vi "String-Array zusammenstutzen.vi"(8 "Array":string[](array[string]), 10 "Anzahl Elemente":i32) -> (0 "Array":string[](array[string]))   [LabVIEW 2020, in "AK-Schnittstelle.lvlib"]
uses:
  AK-Schnittstelle.lvlib
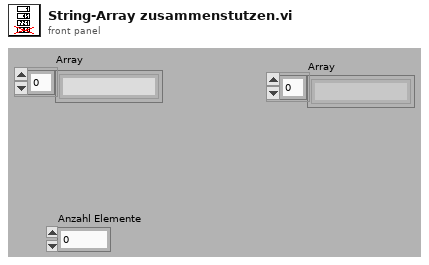
[diagram p1: front panel]
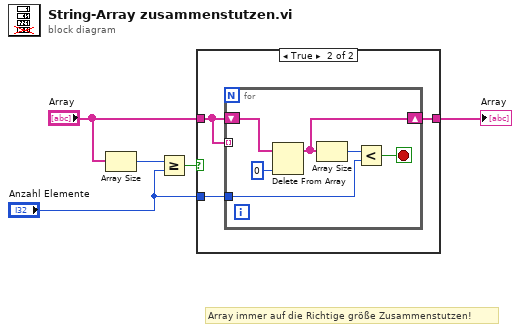
[diagram p0: block diagram]
diagram:
  # "Array immer auf die Richtige größe Zusammenstutzen!"
  n1 = Array Size(array="Array") -> (size(s)=w4:i32)
  n2 = Greater Or Equal?(x=w4, y="Anzahl Elemente") -> (x >= y?=w5:bool)
  n3 = case shown="True" w5 {
    tunnel: "Array" -> [w6 w8]
    tunnel: [w6 w7] -> w1
    tunnel: "Anzahl Elemente" -> [_ w9]
    frame False {
    }
    frame True {
      n4 = for {
        tunnel: w9 -> [w13]
        tunnel: w8 -> [_] mode=indexing
        shift-right: [w10] -> w7
        shift-left: w8 -> [w15]
        stop <- w12 stop-if-true
        n5 = Delete From Array(array=w15, index=0 ("Index")) -> (array with subset deleted=w10:string[])  [unwired: 1 in, 1 out]
        n6 = Array Size(array=w10) -> (size(s)=w14:i32)
        n7 = Less?(x=w14, y=w13) -> (x < y?=w12:bool)
      }
    }
  }
  "Array" <- w1
